vi "StatusMachineEngine.vi"(8 "error in":errorcluster, 11 "Motor Base in":refnum<class "Motor Base.lvclass">) -> (0 "error out":errorcluster, 3 "Motor Base out":refnum<class "Motor Base.lvclass">)   [LabVIEW 2016, in "Motor Base.lvlib" / "Motor Base.lvclass"]
doc: "电机的PDS状态机引擎，调用电机驱动请必须启动此引擎函数。"
uses:
  Motor Base.lvclass
  <vilib>/Platform/TimedLoop/XDataNode/timing_clust.ctl
  <vilib>/Platform/TimedLoop/XDataNode/nitl_modes.ctl
  <vilib>/Platform/TimedLoop/XDataNode/wakeup.ctl
  <vilib>/platform/TimedLoop/XDataNode/XDataNode.xnode
  <vilib>/Platform/TimedLoop/XDataNode/XDNodeRunTimeDep.lvlib
panel:
  # "电机的PDS状态机引擎，调用电机驱动请必须启动此引擎函数。\n孙森\n2017年9月28日20:28:38"
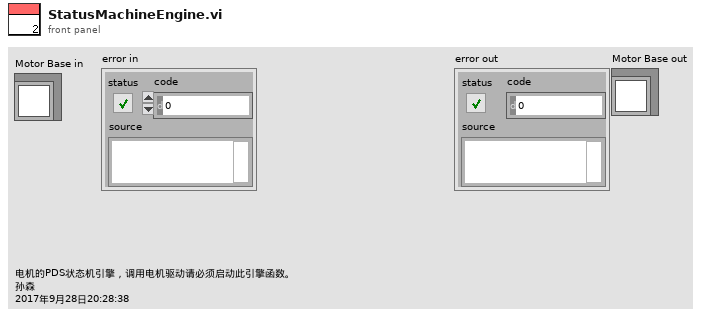
[diagram p1: front panel]
types:
  T1 = typedef "XDNodeRunTimeDep.lvlib/timing_clust.ctl" = cluster{"Expected End [f-1]":u64, "Actual End [f-1]":u64, "Finished Late? [f-1]":bool, "Expected End [i-1]":u64, "Actual End [i-1]":u64, "Finished Late? [i-1]":bool, "Expected Start [i]":u64, "Actual Start [i]":u64, "Expected Start [f]":u64, "Actual Start [f]":u64, "Source Name":string, "Structure Name":string, "Period":i64, "Deadline":i64, "Offset":i64, "Start":i64, "Priority":i32, "Timeout":i32, "Mode":T2, "Wakeup Reason":T3, "Error":errorcluster, "Source Type":string, "Secondary Source Type":string, "Global End Time":u64, "Global Start Time":u64, "Frame Duration":u64, "Iteration Duration":u64, "Assigned CPU":i32, "I/O Scan Engine Mode":u32}
  T2 = typedef "XDNodeRunTimeDep.lvlib/nitl_modes.ctl" = enum32{"No Change", "Process missed periods, maintain original phase", "Discard missed periods, maintain original phase", "Process missed periods, ignore original phase", "Discard missed periods, ignore original phase"}
  T3 = typedef "XDNodeRunTimeDep.lvlib/wakeup.ctl" = enum32{"Normal", "Aborted", "Asynchronous wakeup", "Timing source error", "Timed loop error", "Timeout"}
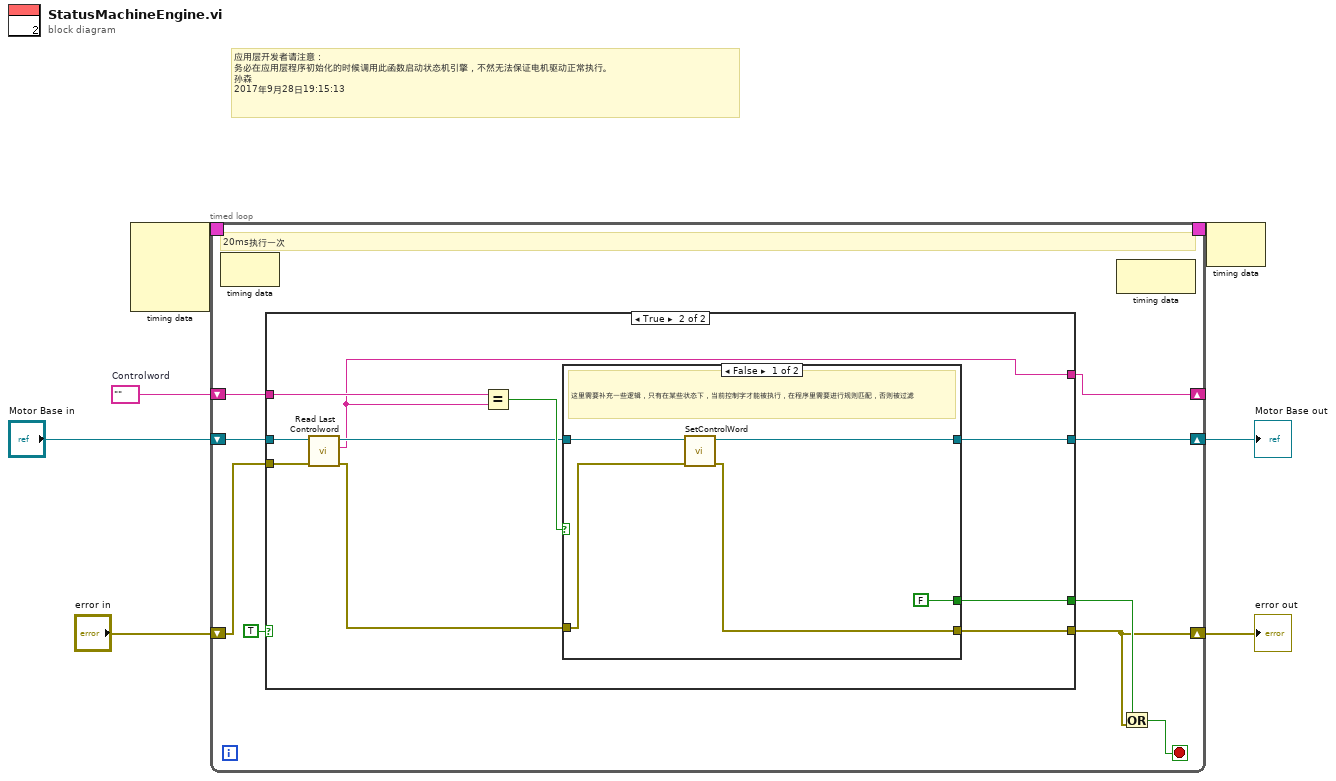
[diagram p0: block diagram]
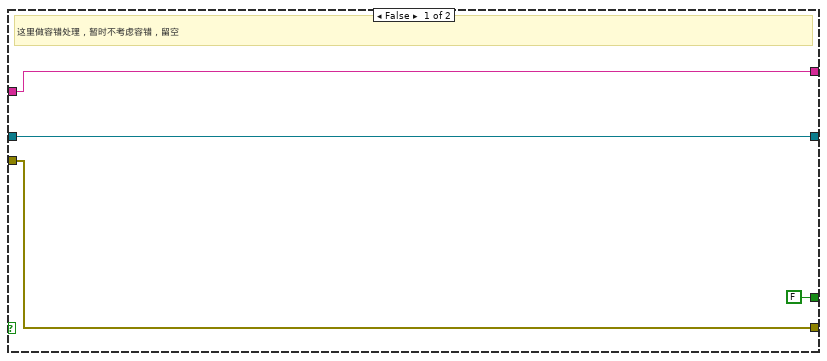
[diagram p2: hidden frame]
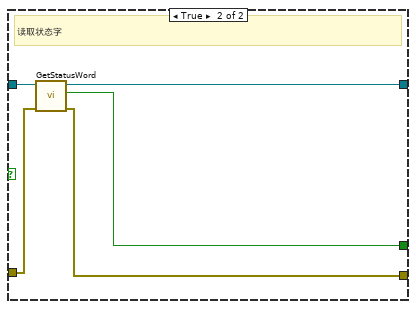
[diagram p3: hidden frame]
diagram:
  w4 = ""  # Controlword
  # "应用层开发者请注意：\n务必在应用层程序初始化的时候调用此函数启动状态机引擎，不然无法保证电机驱动正常执行。\n孙森\n2017年9月28日19:15:13"
  n1 = node-c288() -> (w7:T1)  [unwired: 4 in]
  n2 = timed-loop {
    timing: w7 -> [_]
    timing-out: [_] -> w6
    shift-right: [w14] -> _
    shift-left: w4 -> [w15]
    shift-right: [w13] -> w1
    shift-left: "Motor Base in" -> [w16]
    shift-right: [w9] -> w2
    shift-left: "error in" -> [w8]
    stop <- w11 stop-if-true
    # "20ms执行一次"
    n3 = node-c288() -> ()  [unwired: 1 in, 1 out]
    n4 = case shown="True" TRUE {
      tunnel: w16 -> [w21 w23]
      tunnel: w15 -> [w22 w32]
      tunnel: [w22 w28] -> w14
      tunnel: [w21 w27] -> w13
      tunnel: [w19 w26] -> w9
      tunnel: [FALSE ("Fault") w25] -> w12
      tunnel: w8 -> [w19 w24]
      frame False {
        # "这里做容错处理，暂时不考虑容错，留空"
      }
      frame True {
        n5 = call-dynamic "Read Last Controlword.vi"("error in (no error)"=w24, "Motor Base in"=w23) -> ("error out"=w30:errorcluster, "Controlword"=w28:string, "Motor Base out"=w29:refnum<class "Motor Base.lvclass">)  [unwired: 7 in]
        n6 = Equal?(x=w32, y=w28) -> (x = y?=w31:bool)
        n7 = case shown="False" w31 {
          tunnel: w30 -> [w36 w41]
          tunnel: w29 -> [w37 w42]
          tunnel: [w35 w40] -> w26
          tunnel: [w34 w39] -> w27
          tunnel: [FALSE ("Fault") w38] -> w25
          frame False {
            # "这里需要补充一些逻辑，只有在某些状态下，当前控制字才能被执行，在程序里需要进行规则匹配，否则被过滤"
            n8 = call-dynamic "SetControlWord.vi"("error in (no error)"=w36, "Motor Base in"=w37) -> ("error out"=w35:errorcluster, "Motor Base out"=w34:refnum<class "Motor Base.lvclass">)  [unwired: 8 in]
          }
          frame True {
            # "读取状态字"
            n9 = call-dynamic "GetStatusWord.vi"("error in (no error)"=w41, "Motor Base in"=w42) -> ("error out"=w40:errorcluster, "Fault"=w38:bool, "Motor Base out"=w39:refnum<class "Motor Base.lvclass">)  [unwired: 7 in]
          }
        }
      }
    }
    n10 = node-c288() -> ()  [unwired: 1 in, 1 out]
    n11 = Or(x=w12, y=w9) -> (x .or. y?=w11:bool)
  }
  "error out" <- w2
  "Motor Base out" <- w1
  n12 = node-c288(w6) -> ()  [unwired: 1 out]
